vi "WindowTraceChk.vi"(0 "VISA IN 2":refnum<visa-resource-name>, 1 "Window":i32=1, 2 "Trace":i32=1, 5 "error in":errorcluster) -> (14 "VISA Out 2":refnum<visa-resource-name>, 19 "error out":errorcluster)   [LabVIEW 2018, in "PNA-X.lvlib"]
uses:
  PNA-X.lvlib
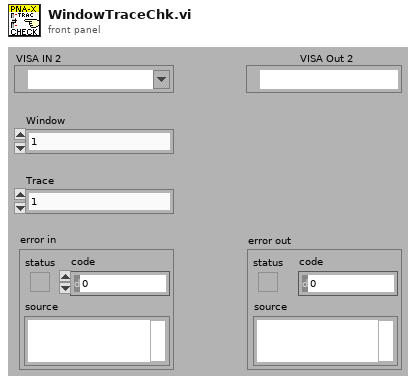
[diagram p1: front panel]
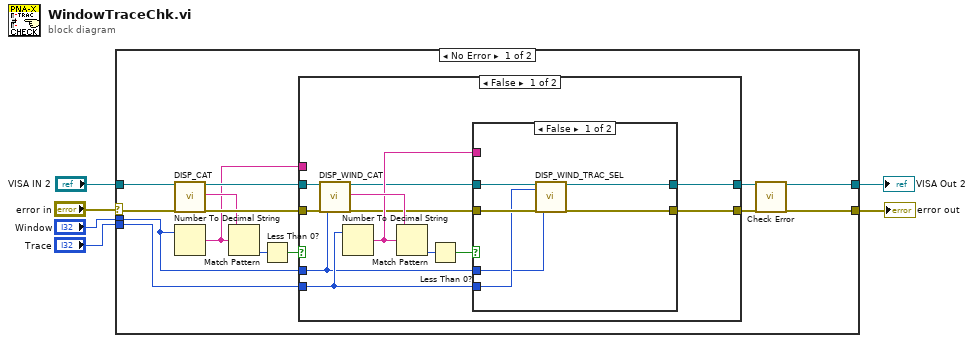
[diagram p0: block diagram]
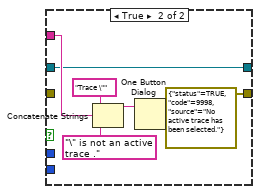
[diagram p2: hidden frame]
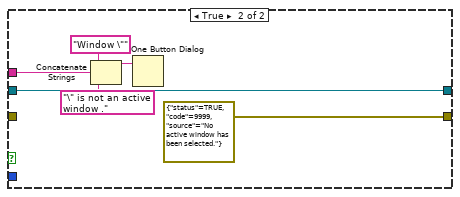
[diagram p3: hidden frame]
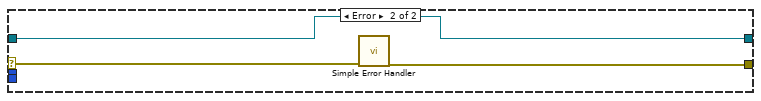
[diagram p4: hidden frame]
diagram:
  n1 = case shown="No Error" "error in" {
    selector: "error in" -> [w17 w53]
    tunnel: [w20 w52] -> w4
    tunnel: "Window" -> [w9 _]
    tunnel: "Trace" -> [w10 _]
    tunnel: "VISA IN 2" -> [w8 w51]
    tunnel: [w7 w51] -> w6
    frame No Error {
      n2 = call "DISP_CAT.vi"("VISA IN"=w8, "error in"=w17) -> ("VISA Out"=w16:refnum<visa-resource-name>, "Data"=w14:string, "error out"=w18:errorcluster)  [unwired: 15 in]
      n3 = Number To Decimal String(number=w9) -> (decimal integer string=w11:string)  [unwired: 1 in]
      n4 = Match Pattern(string=w14, regular expression=w11) -> (offset past match=w13:i32)  [unwired: 1 in, 3 out]
      n5 = Less Than 0?(x=w13) -> (x < 0?=w12:bool)
      n6 = case shown="False" w12 {
        tunnel: [w25 errorcluster {"status"=TRUE, "code"=9999, "source"="No active window has been selected."} ("error out")] -> w19
        tunnel: w18 -> [w32 _]
        tunnel: w16 -> [w31 w50]
        tunnel: [w23 w50] -> w15
        tunnel: w11 -> [_ w49]
        tunnel: w10 -> [w22 _]
        tunnel: w9 -> [w21 _]
        frame False {
          n7 = call "DISP_WIND_CAT.vi"("VISA IN"=w31, "error in"=w32, "Window"=w21) -> ("VISA Out"=w24:refnum<visa-resource-name>, "Data"=w29:string, "error out"=w26:errorcluster)  [unwired: 14 in]
          n8 = Number To Decimal String(number=w22) -> (decimal integer string=w27:string)  [unwired: 1 in]
          n9 = Match Pattern(string=w29, regular expression=w27) -> (offset past match=w30:i32)  [unwired: 1 in, 3 out]
          n10 = Less Than 0?(x=w30) -> (x < 0?=w28:bool)
          n11 = case shown="False" w28 {
            tunnel: w27 -> [_ w41]
            tunnel: w26 -> [w38 _]
            tunnel: [w37 errorcluster {"status"=TRUE, "code"=9998, "source"="No active trace has been selected."} ("error out")] -> w25
            tunnel: w24 -> [w36 w39]
            tunnel: [w35 w39] -> w23
            tunnel: w22 -> [w34 _]
            tunnel: w21 -> [w33 _]
            frame False {
              n12 = call "DISP_WIND_TRAC_SEL.vi"("VISA IN"=w36, "Trace"=w34, "error in"=w38, "Window"=w33) -> ("VISA Out"=w35:refnum<visa-resource-name>, "error out"=w37:errorcluster)  [unwired: 14 in]
            }
            frame True {
              n13 = Concatenate Strings("Trace \"", w41, "\" is not an active trace .") -> (w42:string)
              n14 = One Button Dialog(message=w42) -> ()  [unwired: 1 in, 1 out]
            }
          }
        }
        frame True {
          n15 = Concatenate Strings("Window \"", w49, "\" is not an active window .") -> (w46:string)
          n16 = One Button Dialog(message=w46) -> ()  [unwired: 1 in, 1 out]
        }
      }
      n17 = call "Check Error.vi"("VISA Resource Name"=w15, "error in (no error)"=w19) -> ("dup VISA session"=w7:refnum<visa-resource-name>, "error out"=w20:errorcluster)  [unwired: 16 in]
    }
    frame Error {
      n18 = call <vilib>:"Simple Error Handler.vi"("error in (no error)"=w53) -> ("error out"=w52:errorcluster)  [unwired: 4 in, 4 out]
    }
  }
  "error out" <- w4
  "VISA Out 2" <- w6
